vi "ControllerMain.vi"(9 "AdmittanceCoeffs":T1, 10 "PID gains":T2={"proportional gain (Kc)"=1.0, "integral time (Ti, min)"=0.01, "derivative time (Td, min)"=0.0} {"derivative time (Td, min)" format="%.3f"; "integral time (Ti, min)" format="%.3f"; "proportional gain (Kc)" format="%.3f"}, 11 "?":T3={"ControlFlag"=TRUE, "Fx"=0.0, "Fy"=0.0, "Link1EncPos"=0.0, "Link2EncPos"=0.0, "CurrentX"=0.0, "CurrentY"=0.0, "TargetX"=0.0, "TargetY"=0.0, "DeadZone"=0.0}) -> (0 "Direction 2":bool, 1 "U2":dbl, 2 "Direction1":bool, 3 "U1":dbl)   [LabVIEW 2016, in "controllerLibrary.lvlib"]
uses:
  controllerLibrary.lvlib
  Controls/ControlVariables.ctl
  Controls/AdmittanceGains.ctl
panel:
  out "Theta1":dbl
  out "Theta0":dbl
  out "theta1":dbl
  out "theta0":dbl
  # "Actual"
  # "target"
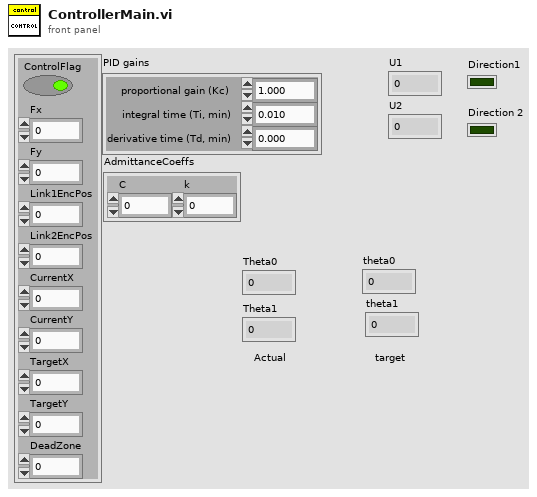
[diagram p1: front panel]
types:
  T1 = typedef "controllerLibrary.lvlib/AdmittanceGains.ctl" = cluster{"C":dbl, "k":dbl}
  T2 = cluster{"proportional gain (Kc)":dbl, "integral time (Ti, min)":dbl, "derivative time (Td, min)":dbl}
  T3 = typedef "controllerLibrary.lvlib/ControlVariables.ctl" = cluster{"ControlFlag":bool, "Fx":dbl, "Fy":dbl, "Link1EncPos":dbl, "Link2EncPos":dbl, "CurrentX":dbl, "CurrentY":dbl, "TargetX":dbl, "TargetY":dbl, "DeadZone":dbl}
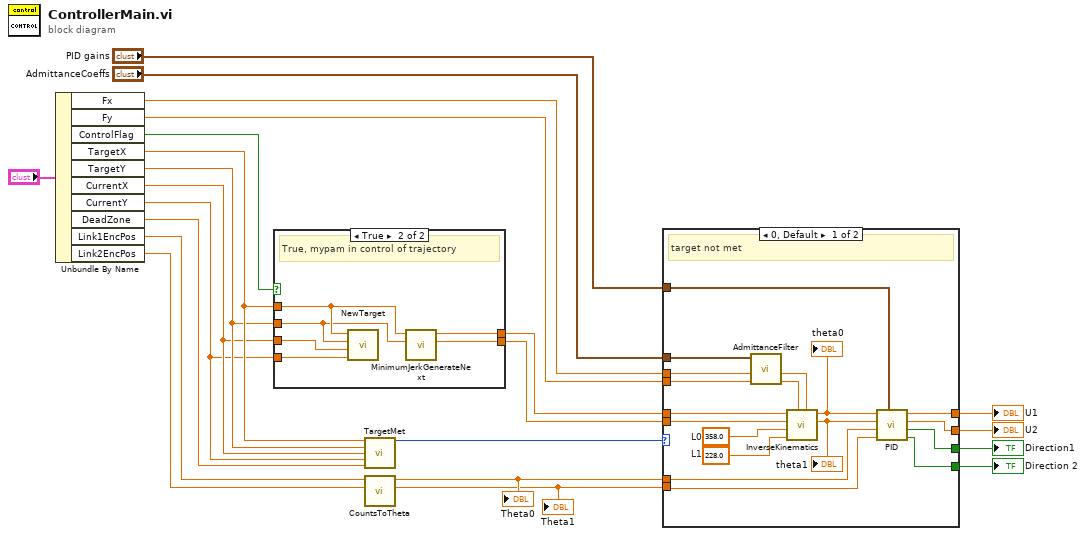
[diagram p0: block diagram]
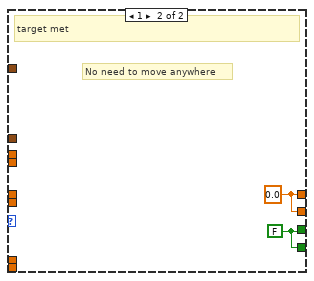
[diagram p2: hidden frame]
diagram:
  n1 = Unbundle By Name("?") -> ("Fx"=w9:dbl, "Fy"=w10:dbl, "ControlFlag"=w21:bool, "TargetX"=w20:dbl, "TargetY"=w19:dbl, "CurrentX"=w18:dbl, "CurrentY"=w17:dbl, "DeadZone"=w16:dbl, "Link1EncPos"=w7:dbl, "Link2EncPos"=w8:dbl)
  n2 = case shown="True" w21 {
    tunnel: w20 -> [w24 w26]
    tunnel: w19 -> [w23 w25]
    tunnel: w18 -> [_ w30]
    tunnel: w17 -> [_ w29]
    tunnel: [w24 w28] -> w14
    tunnel: [w23 w27] -> w13
    frame False {
      # "false, game in control of trajectory"
    }
    frame True {
      # "True, mypam in control of trajectory"
      n3 = call "NewTarget.vi"("Current y"=w29, "Current x"=w30, "Target y"=w25, "Target x"=w26) -> ()  [unwired: 7 in, 1 out]
      n4 = call "MinimumJerkGenerateNext.vi"("Target y"=w25, "Target x"=w26) -> ("yt"=w27:dbl, "xt"=w28:dbl)  [unwired: 8 in]
    }
  }
  n5 = call "TargetMet.vi"("Target x (mm)"=w20, "Target y (mm)"=w19, "Current x (mm)"=w18, "Current y (mm)"=w17, "Dead Zone (mm)"=w16) -> ("out"=w15:i32)  [unwired: 10 in]
  n6 = call "CountsToTheta.vi"("Link2EncPos"=w8, "Link1EncPos"=w7) -> ("Theta1"=w5:dbl, "Theta0"=w6:dbl)  [unwired: 8 in]
  "Theta0" <- w6
  "Theta1" <- w5
  n7 = case shown="0, Default" w15 {
    tunnel: w14 -> [w44 _]
    tunnel: w13 -> [w43 _]
    tunnel: [w42 w50] -> w12
    tunnel: [w41 w50] -> w11
    tunnel: w9 -> [w40 _]
    tunnel: w10 -> [w39 _]
    tunnel: w6 -> [w38 _]
    tunnel: w5 -> [w37 _]
    tunnel: "PID gains" -> [w36 _]
    tunnel: "AdmittanceCoeffs" -> [w35 _]
    tunnel: [w34 w49] -> w2
    tunnel: [w33 w49] -> w1
    frame 0, Default {
      w31 = 228.0  # L1
      w32 = 358.0  # L0
      # "target not met"
      n8 = call "AdmittanceFilter.vi"("Fy"=w39, "Fx"=w40, "AdmittanceCoeffs"=w35) -> ("Delta y"=w46:dbl, "Delta x"=w45:dbl)  [unwired: 7 in]
      n9 = call "InverseKinematics.vi"("deltaX"=w45, "deltaY"=w46, "L1"=w31, "L0"=w32, "Next Y"=w43, "Next X"=w44) -> ("theta1"=w47:dbl, "theta0"=w48:dbl)  [unwired: 4 in]
      "theta0" <- w48
      "theta1" <- w47
      n10 = call "PID.vi"("PID gains"=w36, "current theta1"=w37, "current theta0"=w38, "Des theta1"=w47, "Des theta0"=w48) -> ("Dir2"=w33:bool, "Dir1"=w34:bool, "U2"=w42:dbl, "U1"=w41:dbl)  [unwired: 3 in]
    }
    frame 1 {
      w49 = FALSE
      w50 = 0.0 ("U1")
      # "No need to move anywhere"
      # "target met"
    }
  }
  "U1" <- w11
  "U2" <- w12
  "Direction1" <- w2
  "Direction 2" <- w1
